vi "Format Result Line.vi"(8 "Error in":errorcluster caption="Error in (no error)", 9 "Stats":T1={"Passed"=36, "Failed"=0, "Skipped"=0, "Total"=36}, 10 "Threshold %":dbl, 11 "Rank":string) -> (0 "Error out":errorcluster, 1 "Pass?":bool, 3 "Results Description":string)   [LabVIEW 2023, in "VIA Results Handling.lvlib"]
doc: "Formats a Results Description from the Rank, Threshold %, Stats, and Pass/Fail."
uses:
  VIA Results Handling.lvlib
  Stats Cluster.ctl
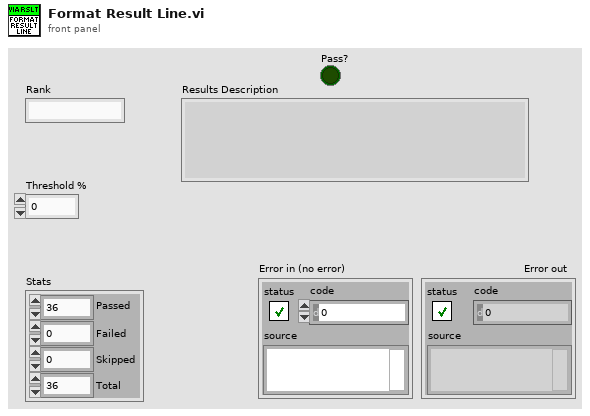
[diagram p1: front panel]
types:
  T1 = typedef "VIA Results Handling.lvlib/Stats Cluster.ctl" = cluster{"Passed":i32, "Failed":i32, "Skipped":i32, "Total":i32}
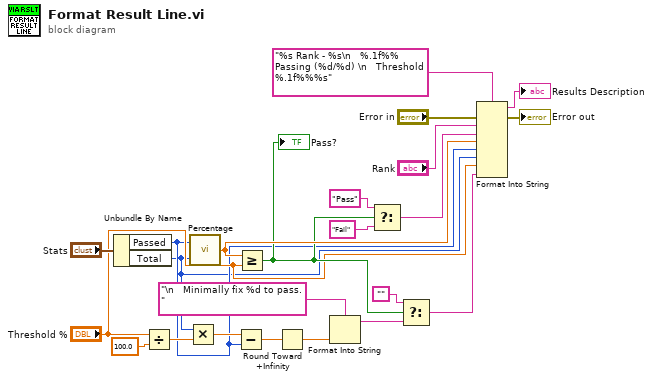
[diagram p0: block diagram]
diagram:
  n1 = Unbundle By Name("Stats") -> ("Passed"=w2:i32, "Total"=w1:i32)
  n2 = Divide(x="Threshold %", y=100.0) -> (x/y=w8:dbl)
  n3 = Multiply(x=w1, y=w8) -> (x*y=w7:dbl)
  n4 = call "Percentage.vi"("A"=w1, "B"=w2) -> ("B/A (%)"=w23:dbl)
  n5 = Subtract(x=w7, y=w2) -> (x-y=w6:dbl)
  n6 = Greater Or Equal?(x=w23, y="Threshold %") -> (x >= y?=w11:bool)
  "Pass?" <- w11
  n7 = Round Toward +Infinity(x=w6) -> (ceil(x): smallest int >= x=w5:dbl)
  n8 = Format Into String(format string="\n   Minimally fix %d to pass.", w5) -> (resulting string=w18:string)  [unwired: 2 in, 1 out]
  n9 = Select(t="Pass", s=w11, f="Fail") -> (s? t:f=w4:string)
  n10 = Select(t="", s=w11, f=w18) -> (s? t:f=w20:string)
  n11 = Format Into String(format string="%s Rank - %s\n   %.1f%% Passing (%d/%d) \n   Threshold %.1f%%%s", error in="Error in", "Rank", w4, w23, w2, w1, "Threshold %", w20) -> (resulting string=→"Results Description":string, error out=→"Error out":errorcluster)  [unwired: 1 in]
